vi "Select Operation.vi"(0 "Guest Manager Model in":refnum<class "Guest Manager Model.lvclass">, 5 "Check-in":bool, 11 "error in (no error)":errorcluster) -> (4 "Guest Manager Model out":refnum<class "Guest Manager Model.lvclass">, 15 "error out":errorcluster)   [LabVIEW 2023, in "Guest Manager Model.lvlib" / "Guest Manager Model.lvclass"]
uses:
  Guest Manager Model.lvclass
  Guest Manager Model.lvclass/Guest Manager Model.ctl
  Guest Manager UI/Guest Manager UI Messages/Select Page Msg/Select Page Msg.lvclass
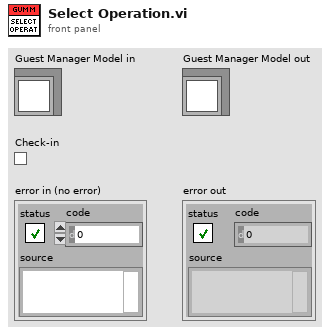
[diagram p1: front panel]
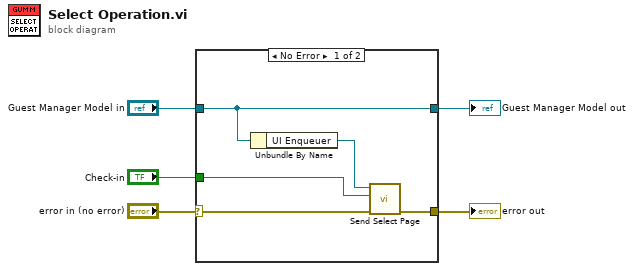
[diagram p0: block diagram]
diagram:
  n1 = case shown="No Error" "error in (no error)" {
    selector: "error in (no error)" -> [w10 w12]
    tunnel: [w9 w12] -> w4
    tunnel: [w8 w11] -> w2
    tunnel: "Guest Manager Model in" -> [w8 w11]
    tunnel: "Check-in" -> [w6 _]
    frame No Error {
      n2 = Unbundle By Name(w8) -> ("UI Enqueuer"=w7:refnum<class "Message Enqueuer.lvclass">)
      n3 = call "Send Select Page.vi"("error in (no error)"=w10, "Check-in"=w6, "Message Enqueuer"=w7) -> ("error out"=w9:errorcluster)  [unwired: 7 in, 1 out]
    }
    frame Error {
    }
  }
  "error out" <- w4
  "Guest Manager Model out" <- w2
